vi "Unguided Move[Conflict].vi"(6 "Power 2":dbl, 7 "Power":dbl=0.6, 8 "error in (no error)":errorcluster, 9 "milliseconds to wait":u32=2500, 10 "refnum name 2":string="Talon1", 11 "refnum name":string="Talon4") -> (0 "error out":errorcluster)   [LabVIEW 2017]
uses:
  <vilib>/Rock Robotics/WPI/ThirdParty/Phoenix-LabVIEW/Motor Controller/Controls/CTRE_Phoenix_MotorControl_ControlMode.ctl
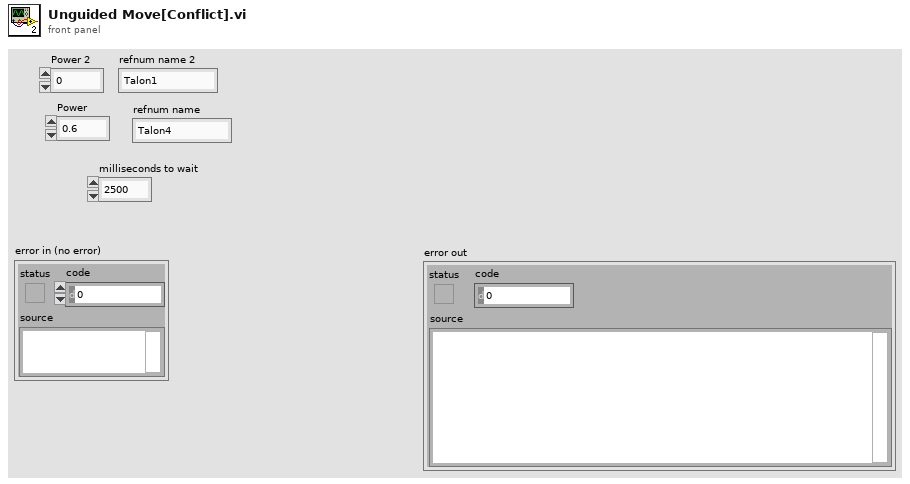
[diagram p1: front panel]
types:
  T1 = typedef "CTRE_Phoenix_MotorControl_ControlMode.ctl" = u16
  T2 = typedef "WPI_MotorControlDeviceRef.ctl" = cluster{"DeviceStatus":errorcluster, "Type":T3, "PWM":cluster{"PWM Channel":T4, "DeadBand":T5}, "CAN":cluster{"Device Number":u8, "SetOutput VI Ref":variant, "GetOutput VI Ref":variant, "Enable VI Ref":variant, "Disable VI Ref":variant, "Data":variant}, "Invert":bool, "DIO PWM":cluster{"PWM \"Enable\" Channel":T4, "DIOChannel":T6, "PWM Rate":dbl}}
  T3 = typedef "WPI_MotorControlType.ctl" = enum16{"PWM", "CAN", "DIO PWM"}
  T4 = typedef "FPGA_DIOPWMChannel.ctl" = enum8{"PWM 0", "PWM 1", "PWM 2", "PWM 3", "PWM 4", "PWM 5", "PWM 6", "PWM 7", "PWM 8", "PWM 9", "PWM MXP 0", "PWM MXP 1", "PWM MXP 2", "PWM MXP 3", "PWM MXP 4", "PWM MXP 5", "PWM MXP 6", "PWM MXP 7", "PWM MXP 8", "PWM MXP 9", "Invalid"}
  T5 = typedef "WPI_PWMDeadband.ctl" = cluster{"Name":string, "maxPositivePwm":i32, "minPositivePwm":i32, "centerPwm":i32, "maxNegativePwm":i32, "minNegativePwm":i32, "angularRange":u16}
  T6 = typedef "FPGA_DIOChannel.ctl" = enum8{"DIO 0", "DIO 1", "DIO 2", "DIO 3", "DIO 4", "DIO 5", "DIO 6", "DIO 7", "DIO 8", "DIO 9", "DIO MXP 0", "DIO MXP 1", "DIO MXP 2", "DIO MXP 3", "DIO MXP 4", "DIO MXP 5", "DIO MXP 6", "DIO MXP 7", "DIO MXP 8", "DIO MXP 9", "DIO MXP 10", "DIO MXP 11", "DIO MXP 12", "DIO MXP 13", "DIO MXP 14", "DIO MXP 15", "SPI Port CS1", "SPI Port CS2", "SPI Port CS3", "SPI Port MISO", "SPI Port MOSI", "Invalid"}
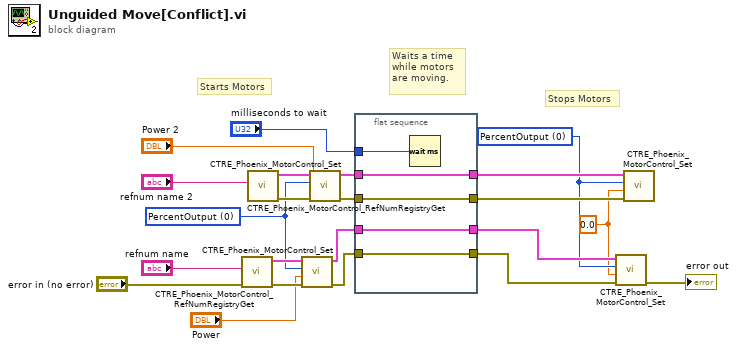
[diagram p0: block diagram]
diagram:
  w6 = 0.0 ("Output")
  w7 = T1 0 items=["PercentOutput"=0, "Position"=1, "Velocity"=2, "Current"=3, "Follower"=5, "MotionProfile"=6, "MotionMagic"=7, "MotionMagicArc"=8, "MotionProfileArc"=10, "Disabled"=15] ("Control Mode")
  w16 = T1 0 items=["PercentOutput"=0, "Position"=1, "Velocity"=2, "Current"=3, "Follower"=5, "MotionProfile"=6, "MotionMagic"=7, "MotionMagicArc"=8, "MotionProfileArc"=10, "Disabled"=15] ("Control Mode")
  # "Stops Motors"
  # "Waits a time \nwhile motors \nare moving."
  # "Starts Motors"
  n1 = call <vilib>:"CTRE_Phoenix_MotorControl_RefNumRegistryGet.vi"("error in (no error)"="error in (no error)", "refnum name"="refnum name") -> ("error out"=w17:errorcluster, "PhoenixMotorControlDevRef"=w18:T2)  [unwired: 8 in]
  n2 = call <vilib>:"CTRE_Phoenix_MotorControl_RefNumRegistryGet.vi"("refnum name"="refnum name 2") -> ("error out"=w20:errorcluster, "PhoenixMotorControlDevRef"=w19:T2)  [unwired: 9 in]
  n3 = call <vilib>:"CTRE_Phoenix_MotorControl_Set.vi"("error in (no error)"=w17, "Output"="Power", "Control Mode"=w16, "PhoenixMotorControlDevRef"=w18) -> ("error out"=w12:errorcluster, "PhoenixMotorControlDevRef"=w13:T2)  [unwired: 6 in]
  n4 = call <vilib>:"CTRE_Phoenix_MotorControl_Set.vi"("error in (no error)"=w20, "Output"="Power 2", "Control Mode"=w16, "PhoenixMotorControlDevRef"=w19) -> ("error out"=w14:errorcluster, "PhoenixMotorControlDevRef"=w15:T2)  [unwired: 6 in]
  n5 = flat-sequence {
    tunnel: w15 -> [w27]
    tunnel: [w27] -> w11
    tunnel: [w26] -> w9
    tunnel: w13 -> [w26]
    tunnel: [w25] -> w8
    tunnel: w12 -> [w25]
    tunnel: w14 -> [w24]
    tunnel: [w24] -> w10
    tunnel: "milliseconds to wait" -> [w23]
    frame #0 {
      n6 = Wait (ms)(milliseconds to wait=w23) -> ()  [unwired: 1 out]
    }
  }
  n7 = call <vilib>:"CTRE_Phoenix_MotorControl_Set.vi"("error in (no error)"=w8, "Output"=w6, "Control Mode"=w7, "PhoenixMotorControlDevRef"=w9) -> ("error out"=→"error out":errorcluster)  [unwired: 6 in, 1 out]
  n8 = call <vilib>:"CTRE_Phoenix_MotorControl_Set.vi"("error in (no error)"=w10, "Output"=w6, "Control Mode"=w7, "PhoenixMotorControlDevRef"=w11) -> ()  [unwired: 6 in, 2 out]
